vi "Difference Comparision.vi"(10 "Image 2":path, 11 "Image 1":path) -> (3 "Difference":dbl)   [LabVIEW 2014, in "Difference Comparision.lvclass"]
uses:
  Difference Comparision.lvclass
  Image Comparison/Image Comparison.lvclass
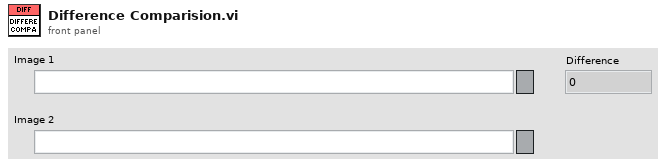
[diagram p1: front panel]
types:
  T1 = typedef "imagedata.ctl" = cluster{"image type":i32, "image depth":i32, "image":u8[], "mask":u8[], "colors":u32[], "Rectangle":cluster{"left":i16, "top":i16, "right":i16, "bottom":i16}}
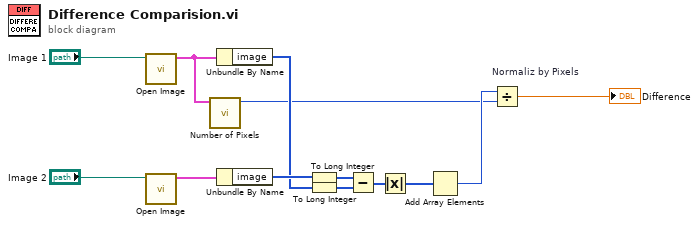
[diagram p0: block diagram]
diagram:
  n1 = call "Open Image.vi"("Image"="Image 1") -> ("image data"=w10:T1)  [unwired: 9 in, 1 out]
  n2 = call "Open Image.vi"("Image"="Image 2") -> ("image data"=w9:T1)  [unwired: 9 in, 1 out]
  n3 = call "Number of Pixels.vi"("image data"=w10) -> ("Number of Pixels"=w1:u64)  [unwired: 10 in]
  n4 = Unbundle By Name(w10) -> ("image"=w4:u8[])
  n5 = Unbundle By Name(w9) -> ("image"=w5:u8[])
  n6 = To Long Integer(number=w5) -> (32bit integer=w7:i32[])
  n7 = To Long Integer(number=w4) -> (32bit integer=w6:i32[])
  n8 = Subtract(x=w7, y=w6) -> (x-y=w8:i32[])
  n9 = Absolute Value(x=w8) -> (abs(x)=w3:i32[])
  n10 = Add Array Elements(numeric array=w3) -> (sum=w2:i32)
  n11 = Divide "Normaliz by Pixels"(x=w2, y=w1) -> (x/y=→"Difference":dbl)
